vi "Convert_Version_ERD.vi"(0 "ERD Data Out":T1[](array[typedef]) {"ERD Number" format="%.0x"}, 11 "Error In":errorcluster) -> (4 "Version":T2, 15 "Error Out":errorcluster)   [LabVIEW 2014]
uses:
  type defs/Version.ctl
  Common/LabVIEW GEA2 Toolkit/LabVIEW_GEA2_Toolkit.lvlibp/type defs/ERD Read Data Out.ctl
  Common/LabVIEW GEA2 Toolkit/LabVIEW_GEA2_Toolkit.lvlibp
panel:
  # "Software Version"
  # "Critical Version"
  # "Non-Critical"
  # "XML Crit Ver"
  # "XML Non-Crit"
  # "Daily Build"
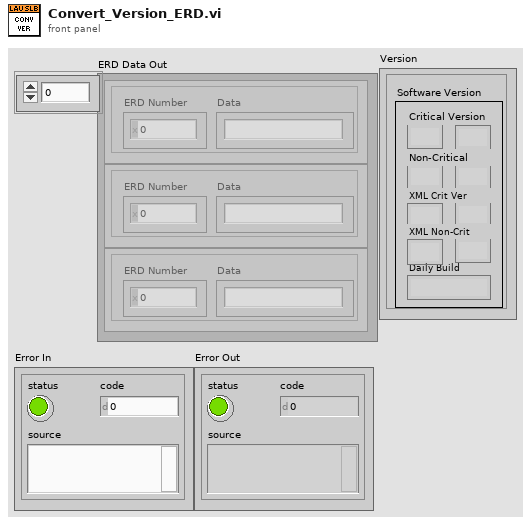
[diagram p1: front panel]
types:
  T1 = typedef "LabVIEW_GEA2_Toolkit.lvlibp/ERD Read Data Out.ctl" = cluster{"ERD Number":u16, "Data":string}
  T2 = typedef "Version.ctl" = cluster{"Critical Major":string, "Critical Minor":string, "Non-Critical Minor":string, "Non-Critical Major":string, "XML Crit Minor":string, "XMLCrit Major":string, "Daily Rev":string, "XML Non-crit Minor":string, "Xml Non-crit Major":string}
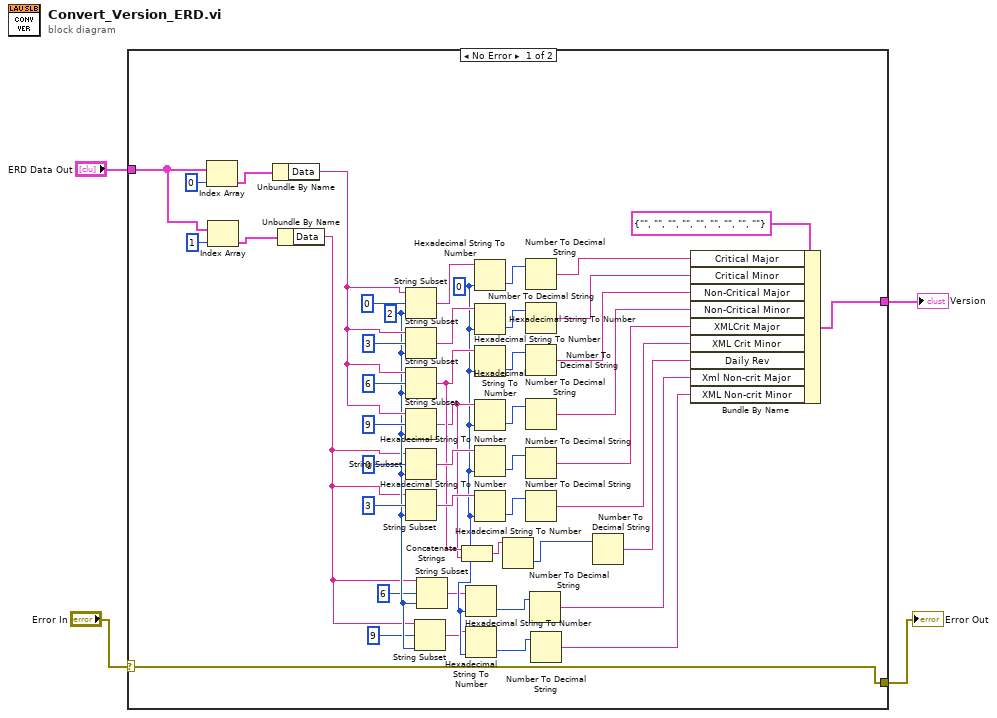
[diagram p0: block diagram]
diagram:
  n1 = case shown="No Error" "Error In" {
    selector: "Error In" -> [w16 w52]
    tunnel: [w16 w52] -> w3
    tunnel: [w29 _] -> w2
    tunnel: "ERD Data Out" -> [w21 _]
    frame No Error {
      w14 = u8 0 ("length (rest)")
      w15 = 2 ("length (rest)")
      n2 = Index Array(array=w21, index=0) -> (element=w20:T1)
      n3 = Index Array(array=w21, index=1) -> (element=w19:T1)
      n4 = Unbundle By Name(w20) -> ("Data"=w17:string)
      n5 = Unbundle By Name(w19) -> ("Data"=w13:string)
      n6 = String Subset(string=w17, offset (0)=0 ("length (rest)"), length (rest)=w15) -> (substring=w50:string)
      n7 = String Subset(string=w17, offset (0)=3 ("length (rest)"), length (rest)=w15) -> (substring=w44:string)
      n8 = String Subset(string=w17, offset (0)=6 ("length (rest)"), length (rest)=w15) -> (substring=w28:string)
      n9 = String Subset(string=w17, offset (0)=9 ("length (rest)"), length (rest)=w15) -> (substring=w27:string)
      n10 = String Subset(string=w13, offset (0)=0 ("length (rest)"), length (rest)=w15) -> (substring=w43:string)
      n11 = String Subset(string=w13, offset (0)=3 ("length (rest)"), length (rest)=w15) -> (substring=w42:string)
      n12 = String Subset(string=w13, offset (0)=9, length (rest)=w15) -> (substring=w11:string)
      n13 = String Subset(string=w13, offset (0)=6, length (rest)=w15) -> (substring=w12:string)
      n14 = Concatenate Strings(w28, w27) -> (w26:string)
      n15 = Hexadecimal String To Number(string=w12, default (0uL)=w14) -> (number=w10:u8)  [unwired: 1 in, 1 out]
      n16 = Hexadecimal String To Number(string=w11, default (0uL)=w14) -> (number=w9:u8)  [unwired: 1 in, 1 out]
      n17 = Hexadecimal String To Number(string=w50, default (0uL)=w14) -> (number=w41:u8)  [unwired: 1 in, 1 out]
      n18 = Hexadecimal String To Number(string=w44, default (0uL)=w14) -> (number=w40:u8)  [unwired: 1 in, 1 out]
      n19 = Hexadecimal String To Number(string=w28, default (0uL)=w14) -> (number=w39:u8)  [unwired: 1 in, 1 out]
      n20 = Hexadecimal String To Number(string=w27, default (0uL)=w14) -> (number=w38:u8)  [unwired: 1 in, 1 out]
      n21 = Hexadecimal String To Number(string=w43, default (0uL)=w14) -> (number=w37:u8)  [unwired: 1 in, 1 out]
      n22 = Hexadecimal String To Number(string=w42, default (0uL)=w14) -> (number=w36:u8)  [unwired: 1 in, 1 out]
      n23 = Hexadecimal String To Number(string=w26) -> (number=w25:u32)  [unwired: 2 in, 1 out]
      n24 = Number To Decimal String(number=w41) -> (decimal integer string=w30:string)  [unwired: 1 in]
      n25 = Number To Decimal String(number=w40) -> (decimal integer string=w31:string)  [unwired: 1 in]
      n26 = Number To Decimal String(number=w39) -> (decimal integer string=w32:string)  [unwired: 1 in]
      n27 = Number To Decimal String(number=w38) -> (decimal integer string=w33:string)  [unwired: 1 in]
      n28 = Number To Decimal String(number=w37) -> (decimal integer string=w34:string)  [unwired: 1 in]
      n29 = Number To Decimal String(number=w36) -> (decimal integer string=w35:string)  [unwired: 1 in]
      n30 = Number To Decimal String(number=w10) -> (decimal integer string=w8:string)  [unwired: 1 in]
      n31 = Number To Decimal String(number=w9) -> (decimal integer string=w7:string)  [unwired: 1 in]
      n32 = Number To Decimal String(number=w25) -> (decimal integer string=w24:string)  [unwired: 1 in]
      n33 = Bundle By Name(cluster=T2 {"Critical Major"="", "Critical Minor"="", "Non-Critical Minor"="", "Non-Critical Major"="", "XML Crit Minor"="", "XMLCrit Major"="", "Daily Rev"="", "XML Non-crit Minor"="", "Xml Non-crit Major"=""} ("Version"), "Critical Major"=w30, "Critical Minor"=w31, "Non-Critical Major"=w32, "Non-Critical Minor"=w33, "XMLCrit Major"=w34, "XML Crit Minor"=w35, "Daily Rev"=w24, "Xml Non-crit Major"=w8, "XML Non-crit Minor"=w7) -> (w29:T2)
    }
    frame Error {
    }
  }
  "Error Out" <- w3
  "Version" <- w2
